vi "REV Robotics Analog Pressure Sensor - Voltage to Pressure.vi"(5 "Averaging Size":i32=20, 9 "Voltage (V)":dbl) -> (3 "Pressure (PSI)":dbl)   [LabVIEW 2015]
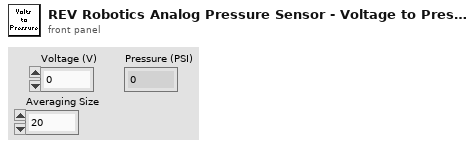
[diagram p1: front panel]
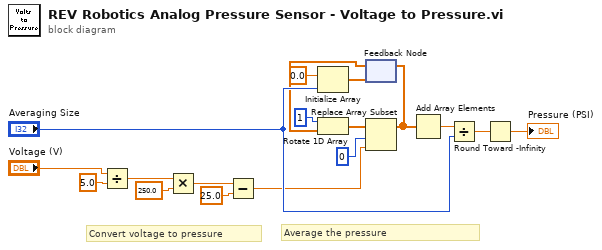
[diagram p0: block diagram]
diagram:
  # "Average the pressure"
  # "Convert voltage to pressure"
  n1 = Divide(x="Voltage (V)", y=5.0) -> (x/y=w5:dbl)
  n2 = Multiply(x=w5, y=250.0) -> (x*y=w3:dbl)
  n3 = Subtract(x=w3, y=25.0) -> (x-y=w7:dbl)
  n4 = Initialize Array(0.0, "Averaging Size") -> (w13:dbl[])
  n5 = feedback #1(w13) -> (w14:dbl[])
  n6 = Rotate 1D Array(1:w14, 2:1 ("n")) -> (0:w15:dbl[])
  n7 = Replace Array Subset(array=w15, new element=w7, index=0) -> (w12:dbl[])
  n8 = feedback-in #1(w12) -> ()
  n9 = Add Array Elements(numeric array=w12) -> (sum=w8:dbl)
  n10 = Divide(x=w8, y="Averaging Size") -> (x/y=w10:dbl)
  n11 = Round Toward -Infinity(1:w10) -> (0:→"Pressure (PSI)":dbl)
